vi "strike_distance.vi"(2 "Numeric":dbl, 3 "reference":refnum<vi>) -> (0 "Strike distance Km":dbl, 1 "kV/m tampone":dbl)   [LabVIEW 2010]
panel:
  out "Inversione segno ?":bool
  out "Post_fulmine":string
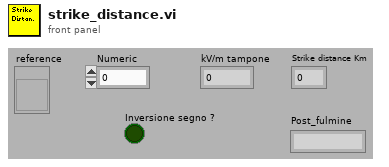
[diagram p1: front panel]
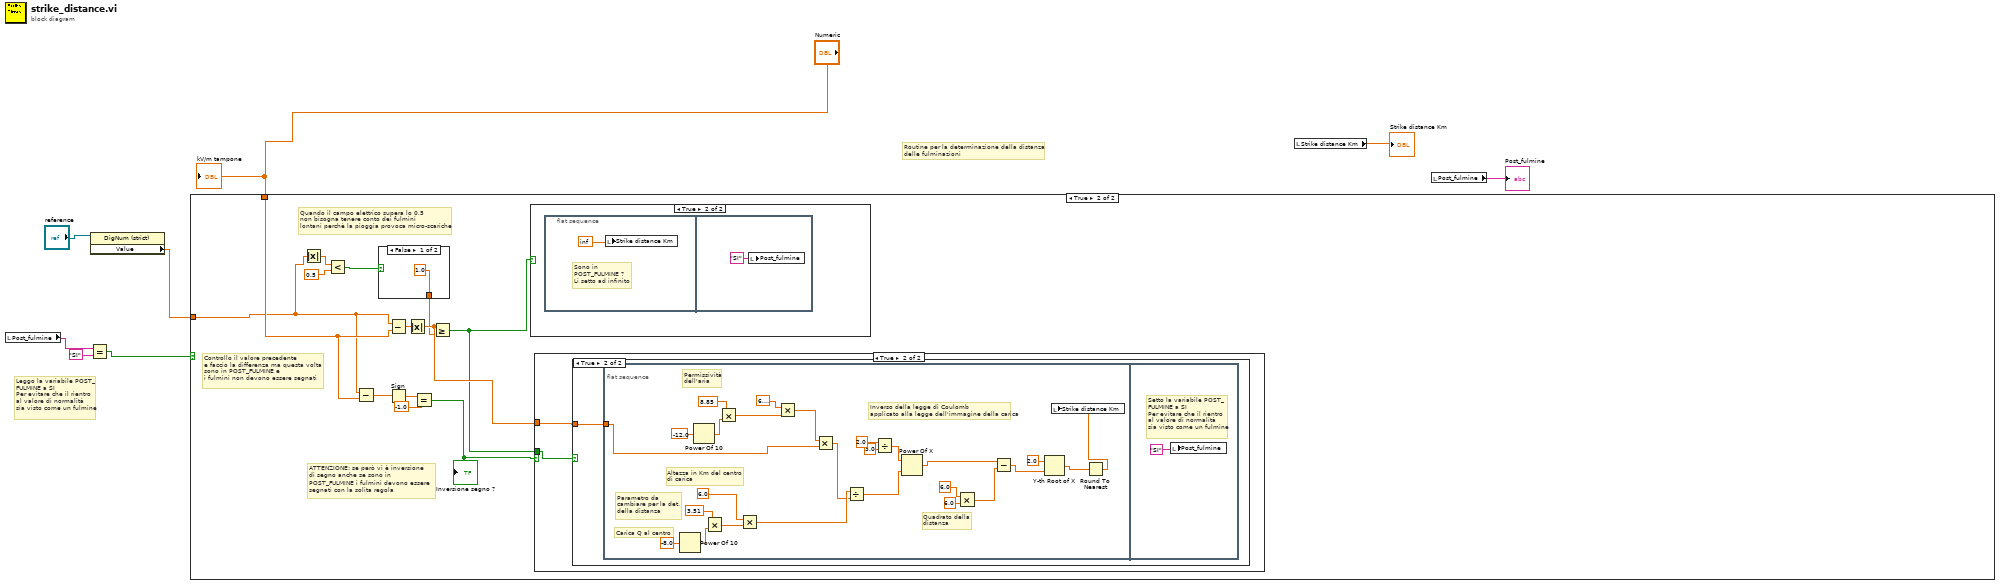
[diagram p0: block diagram]
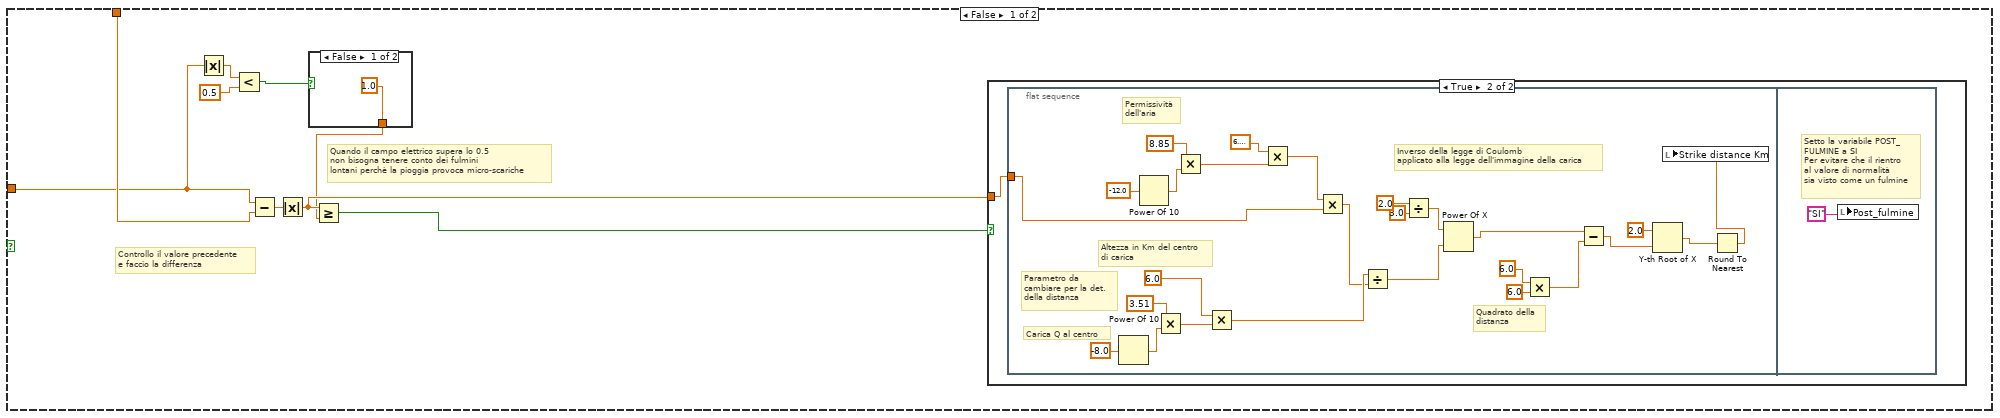
[diagram p2: hidden frame]
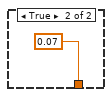
[diagram p3: hidden frame]
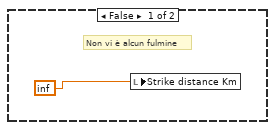
[diagram p4: hidden frame]
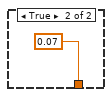
[diagram p5: hidden frame]
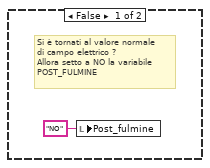
[diagram p8: hidden frame]
diagram:
  # "Leggo la variabile POST_\nFULMINE a SI\nPer evitare che il rientro\nal valore di normalità\nsia visto come un fulmine"
  # "Routine per la determinazione della distanza\ndelle fulminazioni"
  n1 = local read "Post_fulmine"() -> (w5:string)
  n2 = Equal?(x=w5, y="SI") -> (x = y?=w3:bool)
  n3 = property class="DigNum (strict)"(reference="reference") -> ("Value"=w1:dbl)  [unwired: 1 in, 2 out]
  n4 = case shown="True" w3 {
    tunnel: "Numeric" -> [w14 w57]
    tunnel: w1 -> [w9 w50]
    frame False {
      # "Quando il campo elettrico supera lo 0.5\nnon bisogna tenere conto dei fulmini\nlontani perchè la pioggia provoca micro-scariche"
      # "Controllo il valore precedente\ne faccio la differenza"
      n5 = Absolute Value(x=w9) -> (abs(x)=w11:dbl)
      n6 = Less?(x=w11, y=0.5) -> (x < y?=w12:bool)
      n7 = Subtract(x=w9, y=w14) -> (x-y=w16:dbl)
      n8 = Absolute Value(x=w16) -> (abs(x)=w17:dbl)
      n9 = case shown="False" w12 {
        tunnel: [1.0 ("y") 0.07 ("y")] -> w10
        frame False {
        }
        frame True {
        }
      }
      n10 = Greater Or Equal?(x=w17, y=w10) -> (x >= y?=w15:bool)
      n11 = case shown="True" w15 {
        tunnel: w17 -> [_ w21]
        frame False {
          # "Non vi è alcun fulmine"
          n12 = local write "Strike distance Km"(inf) -> ()
        }
        frame True {
          n13 = flat-sequence {
            tunnel: w21 -> [w23]
            frame #0 {
              # "Parametro da\ncambiare per la det.\ndella distanza"
              # "Inverso della legge di Coulomb\napplicato alla legge dell'immagine della carica"
              # "Quadrato della\ndistanza"
              # "Permissività\ndell'aria"
              # "Carica Q al centro"
              # "Altezza in Km del centro\ndi carica"
              n14 = Power Of 10(x=-8.0) -> (10^x=w45:dbl)
              n15 = Power Of 10(x=-12.0) -> (10^x=w42:dbl)
              n16 = Multiply(x=3.51, y=w45) -> (x*y=w38:dbl)
              n17 = Multiply(x=8.85, y=w42) -> (x*y=w40:dbl)
              n18 = Multiply(x=6.0, y=w38) -> (x*y=w37:dbl)
              n19 = Multiply(x=6.283185307179586, y=w40) -> (x*y=w39:dbl)
              n20 = Multiply(x=w39, y=w23) -> (x*y=w36:dbl)
              n21 = Divide(x=w37, y=w36) -> (x/y=w35:dbl)
              n22 = Divide(x=2.0, y=3.0) -> (x/y=w32:dbl)
              n23 = Power Of X(1:w35, 2:w32) -> (0:w31:dbl)
              n24 = Multiply(x=6.0, y=6.0) -> (x*y=w28:dbl)
              n25 = Subtract(x=w31, y=w28) -> (x-y=w30:dbl)
              n26 = Y-th Root of X(1:w30, 2:2.0 ("y")) -> (0:w24:dbl)
              n27 = Round To Nearest(number=w24) -> (nearest integer value=w22:dbl)
              n28 = local write "Strike distance Km"(w22) -> ()
            }
            frame #1 {
              # "Setto la variabile POST_\nFULMINE a SI\nPer evitare che il rientro\nal valore di normalità\nsia visto come un fulmine"
              n29 = local write "Post_fulmine"("SI") -> ()
            }
          }
        }
      }
    }
    frame True {
      # "Quando il campo elettrico supera lo 0.5\nnon bisogna tenere conto dei fulmini\nlontani perchè la pioggia provoca micro-scariche"
      # "ATTENZIONE: se però vi è inversione \ndi segno anche se sono in\nPOST_FULMINE i fulmini devono essere \nsegnati con la solita regola"
      # "Controllo il valore precedente\ne faccio la differenza ma questa volta\nsono in POST_FULMINE e\ni fulmini non devono essere segnati"
      n30 = Absolute Value(x=w50) -> (abs(x)=w49:dbl)
      n31 = Less?(x=w49, y=0.5) -> (x < y?=w52:bool)
      n32 = Subtract(x=w50, y=w57) -> (x-y=w58:dbl)
      n33 = case shown="False" w52 {
        tunnel: [1.0 ("y") 0.07 ("y")] -> w51
        frame False {
        }
        frame True {
        }
      }
      n34 = Subtract(x=w50, y=w57) -> (x-y=w61:dbl)
      n35 = Sign(1:w58) -> (0:w60:dbl)
      n36 = Absolute Value(x=w61) -> (abs(x)=w56:dbl)
      n37 = Equal?(x=w60, y=-1.0) -> (x = y?=w55:bool)
      "Inversione segno ?" <- w55
      n38 = Greater Or Equal?(x=w56, y=w51) -> (x >= y?=w54:bool)
      n39 = case shown="True" w54 {
        frame False {
          # "Si è tornati al valore normale\ndi campo elettrico ?\nAllora setto a NO la variabile\nPOST_FULMINE"
          n40 = local write "Post_fulmine"("NO" ("Post_fulmine")) -> ()
        }
        frame True {
          n41 = flat-sequence {
            frame #0 {
              # "Sono in \nPOST_FULMINE ?\nLi setto ad infinito"
              n42 = local write "Strike distance Km"(inf) -> ()
            }
            frame #1 {
              n43 = local write "Post_fulmine"("SI" ("Post_fulmine")) -> ()
            }
          }
        }
      }
      n44 = case shown="True" w55 {
        tunnel: w56 -> [_ w65]
        tunnel: w54 -> [_ w64]
        frame False {
        }
        frame True {
          n45 = case shown="True" w64 {
            tunnel: w65 -> [_ w66]
            frame False {
            }
            frame True {
              n46 = flat-sequence {
                tunnel: w66 -> [w68]
                frame #0 {
                  # "Parametro da\ncambiare per la det.\ndella distanza"
                  # "Inverso della legge di Coulomb\napplicato alla legge dell'immagine della carica"
                  # "Quadrato della\ndistanza"
                  # "Permissività\ndell'aria"
                  # "Carica Q al centro"
                  # "Altezza in Km del centro\ndi carica"
                  n47 = Power Of 10(x=-8.0) -> (10^x=w90:dbl)
                  n48 = Power Of 10(x=-12.0) -> (10^x=w87:dbl)
                  n49 = Multiply(x=3.51, y=w90) -> (x*y=w83:dbl)
                  n50 = Multiply(x=8.85, y=w87) -> (x*y=w85:dbl)
                  n51 = Multiply(x=6.0, y=w83) -> (x*y=w82:dbl)
                  n52 = Multiply(x=6.283185307179586, y=w85) -> (x*y=w84:dbl)
                  n53 = Multiply(x=w84, y=w68) -> (x*y=w81:dbl)
                  n54 = Divide(x=w82, y=w81) -> (x/y=w80:dbl)
                  n55 = Divide(x=2.0, y=3.0) -> (x/y=w77:dbl)
                  n56 = Power Of X(1:w80, 2:w77) -> (0:w76:dbl)
                  n57 = Multiply(x=6.0, y=6.0) -> (x*y=w73:dbl)
                  n58 = Subtract(x=w76, y=w73) -> (x-y=w75:dbl)
                  n59 = Y-th Root of X(1:w75, 2:2.0 ("y")) -> (0:w69:dbl)
                  n60 = Round To Nearest(number=w69) -> (nearest integer value=w67:dbl)
                  n61 = local write "Strike distance Km"(w67) -> ()
                }
                frame #1 {
                  # "Setto la variabile POST_\nFULMINE a SI\nPer evitare che il rientro\nal valore di normalità\nsia visto come un fulmine"
                  n62 = local write "Post_fulmine"("SI") -> ()
                }
              }
            }
          }
        }
      }
    }
  }
  n63 = local read "Strike distance Km"() -> (→"Strike distance Km":dbl)
  n64 = local read "Post_fulmine"() -> (→"Post_fulmine":string)
  "kV/m tampone" <- "Numeric"
